vi "AVQ8347 Wavelike Data.vi"(0 "VISA Session":refnum<visa-resource-name>, 1 "Axis Select":T1(ring), 5 "Error In":errorcluster) -> (14 "Copy VISA Session":refnum<visa-resource-name>, 15 "Return All Data":string, 16 "Wavelike Data":dbl[](array[numeric]) format="%.12f", 17 "Return Data Bytes":u16, 19 "Error Out":errorcluster)   [LabVIEW 2020]
doc: "This function returns the wavelike data value\n\n(NEC-PC Mode Data is Return All Data Only)"
panel:
  out "CntWk":u16
  out "String Work":string
  # "Wavelike Data"
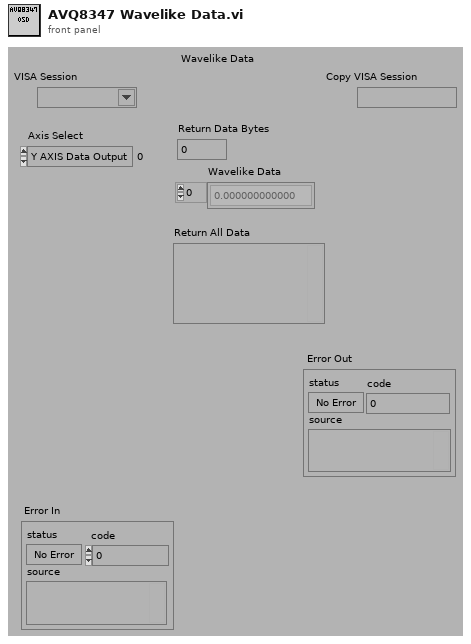
[diagram p1: front panel]
types:
  T1 = enum16{"Y AXIS Data Output", "X AXIS Data Output"}
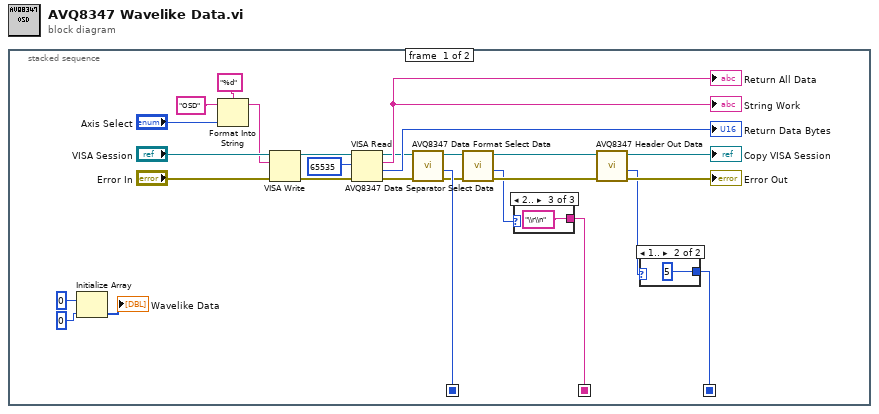
[diagram p0: block diagram]
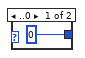
[diagram p2: hidden frame]
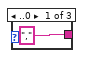
[diagram p3: hidden frame]
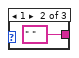
[diagram p4: hidden frame]
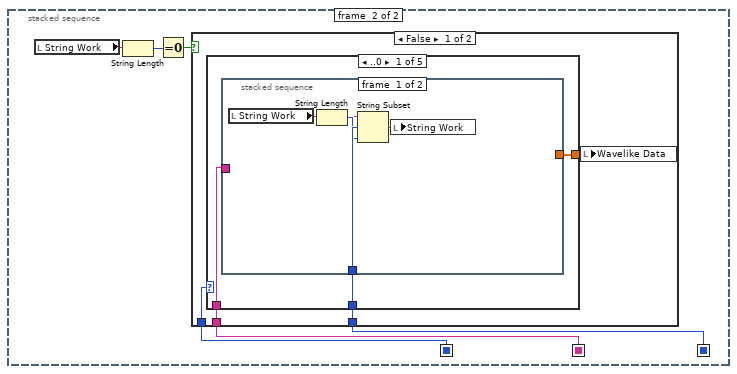
[diagram p5: hidden frame]
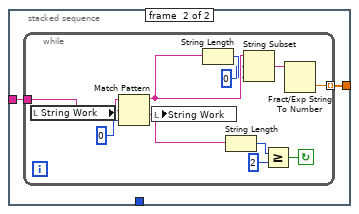
[diagram p6: hidden frame]
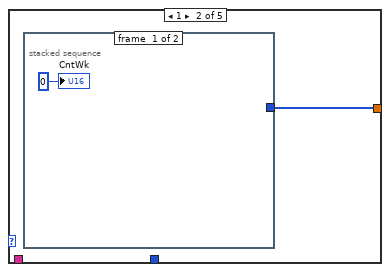
[diagram p7: hidden frame]
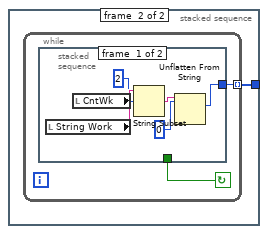
[diagram p8: hidden frame]
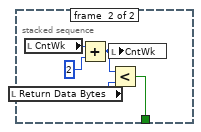
[diagram p9: hidden frame]
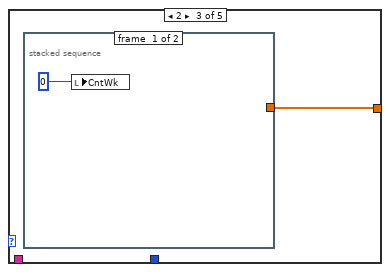
[diagram p10: hidden frame]
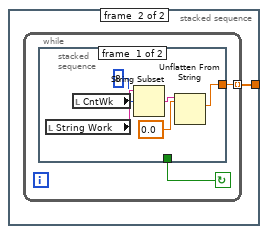
[diagram p11: hidden frame]
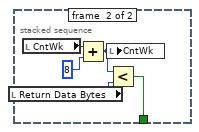
[diagram p12: hidden frame]
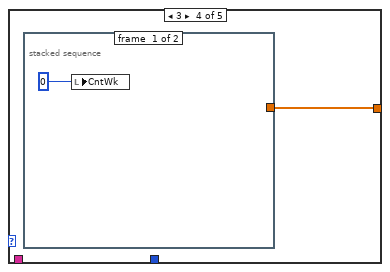
[diagram p13: hidden frame]
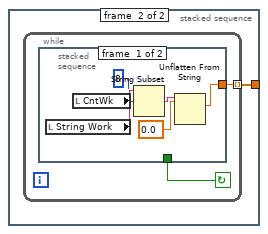
[diagram p14: hidden frame]
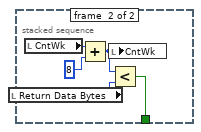
[diagram p15: hidden frame]
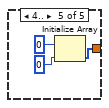
[diagram p16: hidden frame]
diagram:
  n1 = stacked-sequence {
    seq-local: [w17 _] -> [_ w35]
    seq-local: [w22 _] -> [_ w33]
    seq-local: [w11 _] -> [_ w34]
    frame #0 {
      n2 = Initialize Array(0, 0) -> (→"Wavelike Data":i32[])
      n3 = Format Into String(format string="%d", initial string="OSD", "Axis Select") -> (resulting string=w13:string)  [unwired: 1 in, 1 out]
      n4 = VISA Write(VISA resource name="VISA Session", write buffer=w13, error in (no error)="Error In") -> (VISA resource name out=w23:refnum<visa-resource-name>, error out=w24:errorcluster)  [unwired: 1 out]
      n5 = VISA Read(VISA resource name=w23, byte count=65535, error in (no error)=w24) -> (VISA resource name out=w2:refnum<visa-resource-name>, read buffer=→"String Work" →"Return All Data":string, return count=→"Return Data Bytes":u32, error out=w1:errorcluster)
      n6 = call "AVQ8347 Data Format Select Data.vi"("Error In"=w1, "VISA Session"=w2) -> ("Error Out"=w10:errorcluster, "Data Format Select Value"=w11:u16, "Copy VISA Session"=w12:refnum<visa-resource-name>)  [unwired: 6 in, 1 out]
      n7 = call "AVQ8347 Data Separator Select Data.vi"("Error In"=w10, "VISA Session"=w12) -> ("Error Out"=w9:errorcluster, "Data Separrator Select Value"=w7:u16, "Copy VISA Session"=w8:refnum<visa-resource-name>)  [unwired: 6 in, 1 out]
      n8 = case shown="2.." w7 {
        tunnel: ["," " " "\\r\\n"] -> w17
        frame ..0 {
        }
        frame 1 {
        }
        frame 2.. {
        }
      }
      n9 = call "AVQ8347 Header Out Data.vi"("Error In"=w9, "VISA Session"=w8) -> ("Error Out"=→"Error Out":errorcluster, "Header Data Out Control Value"=w4:u16, "Copy VISA Session"=→"Copy VISA Session":refnum<visa-resource-name>)  [unwired: 6 in, 1 out]
      n10 = case shown="1.." w4 {
        tunnel: [0 5] -> w22
        frame ..0 {
        }
        frame 1.. {
        }
      }
    }
    frame #1 {
      n11 = local read "String Work"() -> (w38:string)
      n12 = String Length(string=w38) -> (length=w37:i32)
      n13 = Equal To 0?(x=w37) -> (x = 0?=w36:bool)
      n14 = case shown="False" w36 {
        tunnel: w35 -> [w42 _]
        tunnel: w34 -> [w41 _]
        tunnel: w33 -> [w40 _]
        frame False {
          n15 = case shown="..0" w41 {
            tunnel: w42 -> [w45 _ _ _ _]
            tunnel: w40 -> [w44 _ _ _ _]
            tunnel: [w43 w64 w80 w96 w112] -> w39
            frame ..0 {
              n16 = stacked-sequence {
                tunnel: w44 -> [w49 _]
                tunnel: w45 -> [_ w51]
                tunnel: [_ w50] -> w43
                frame #0 {
                  n17 = local read "String Work"() -> (w47:string)
                  n18 = String Length(string=w47) -> (length=w48:i32)
                  n19 = String Subset(string=w47, offset (0)=w49, length (rest)=w48) -> (substring=w46:string)
                  n20 = local write "String Work"(w46) -> ()
                }
                frame #1 {
                  n21 = while {
                    tunnel: [w58] -> w50 mode=indexing
                    tunnel: w51 -> [w57]
                    stop <- w54 continue-if-true
                    n22 = local read "String Work"() -> (w59:string)
                    n23 = Match Pattern(string=w59, regular expression=w57, offset (0)=0) -> (before substring=w62:string, after substring=w60:string)  [unwired: 2 out]
                    n24 = local write "String Work"(w60) -> ()
                    n25 = String Length(string=w62) -> (length=w61:i32)
                    n26 = String Length(string=w60) -> (length=w55:i32)
                    n27 = String Subset(string=w62, offset (0)=0, length (rest)=w61) -> (substring=w63:string)
                    n28 = Greater Or Equal?(x=w55, y=2) -> (x >= y?=w54:bool)
                    n29 = Fract/Exp String To Number(string=w63) -> (number=w58:dbl)  [unwired: 3 in, 1 out]
                  }
                }
              }
            }
            frame 1 {
              n30 = stacked-sequence {
                tunnel: [_ w66] -> w64
                frame #0 {
                  "CntWk" <- 0
                }
                frame #1 {
                  n31 = while {
                    tunnel: [w67] -> w66 mode=indexing
                    stop <- w68 continue-if-true
                    n32 = stacked-sequence {
                      tunnel: [_ w77] -> w68
                      tunnel: [w71 _] -> w67
                      frame #0 {
                        n33 = local read "String Work"() -> (w74:string)
                        n34 = local read "CntWk"() -> (w73:u16)
                        n35 = String Subset(string=w74, offset (0)=w73, length (rest)=2) -> (substring=w72:string)
                        n36 = Unflatten From String(type=u16 0, binary string=w72) -> (value=w71:u16)  [unwired: 3 in, 2 out]
                      }
                      frame #1 {
                        n37 = local read "Return Data Bytes"() -> (w75:u16)
                        n38 = local read "CntWk"() -> (w79:u16)
                        n39 = Add(x=w79, y=2) -> (x+y=w76:i32)
                        n40 = local write "CntWk"(w76) -> ()
                        n41 = Less?(x=w76, y=w75) -> (x < y?=w77:bool)
                      }
                    }
                  }
                }
              }
            }
            frame 2 {
              n42 = stacked-sequence {
                tunnel: [_ w82] -> w80
                frame #0 {
                  n43 = local write "CntWk"(0) -> ()
                }
                frame #1 {
                  n44 = while {
                    tunnel: [w83] -> w82 mode=indexing
                    stop <- w84 continue-if-true
                    n45 = stacked-sequence {
                      tunnel: [_ w93] -> w84
                      tunnel: [w87 _] -> w83
                      frame #0 {
                        n46 = local read "String Work"() -> (w90:string)
                        n47 = local read "CntWk"() -> (w89:u16)
                        n48 = String Subset(string=w90, offset (0)=w89, length (rest)=8) -> (substring=w88:string)
                        n49 = Unflatten From String(type=0.0, binary string=w88) -> (value=w87:dbl)  [unwired: 3 in, 2 out]
                      }
                      frame #1 {
                        n50 = local read "Return Data Bytes"() -> (w91:u16)
                        n51 = local read "CntWk"() -> (w95:u16)
                        n52 = Add(x=w95, y=8) -> (x+y=w92:i32)
                        n53 = local write "CntWk"(w92) -> ()
                        n54 = Less?(x=w92, y=w91) -> (x < y?=w93:bool)
                      }
                    }
                  }
                }
              }
            }
            frame 3 {
              n55 = stacked-sequence {
                tunnel: [_ w98] -> w96
                frame #0 {
                  n56 = local write "CntWk"(0) -> ()
                }
                frame #1 {
                  n57 = while {
                    tunnel: [w99] -> w98 mode=indexing
                    stop <- w100 continue-if-true
                    n58 = stacked-sequence {
                      tunnel: [_ w109] -> w100
                      tunnel: [w103 _] -> w99
                      frame #0 {
                        n59 = local read "String Work"() -> (w106:string)
                        n60 = local read "CntWk"() -> (w105:u16)
                        n61 = String Subset(string=w106, offset (0)=w105, length (rest)=8) -> (substring=w104:string)
                        n62 = Unflatten From String(type=sgl 0.0, binary string=w104) -> (value=w103:sgl)  [unwired: 3 in, 2 out]
                      }
                      frame #1 {
                        n63 = local read "Return Data Bytes"() -> (w107:u16)
                        n64 = local read "CntWk"() -> (w111:u16)
                        n65 = Add(x=w111, y=8) -> (x+y=w108:i32)
                        n66 = local write "CntWk"(w108) -> ()
                        n67 = Less?(x=w108, y=w107) -> (x < y?=w109:bool)
                      }
                    }
                  }
                }
              }
            }
            frame 4.. {
              n68 = Initialize Array(0, 0) -> (w112:i32[])
            }
          }
          n69 = local write "Wavelike Data"(w39) -> ()
        }
        frame True {
        }
      }
    }
  }
